vi "F_to_C.vi"(10 "숫자형 입력":dbl) -> (1 "숫자형 출력":dbl)   [LabVIEW 2018]
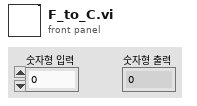
[diagram p1: front panel]
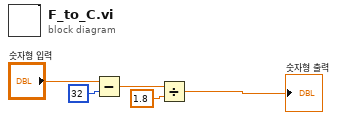
[diagram p0: block diagram]
diagram:
  n1 = Subtract(x="숫자형 입력", y=32) -> (x-y=w4:dbl)
  n2 = Divide(x=w4, y=1.8) -> (x/y=→"숫자형 출력":dbl)
